vi "Read enemyGoalPosition.vi"(8 "error in (no error)":errorcluster, 11 "Field in":refnum<class "Field.lvclass">) -> (0 "error out":errorcluster, 2 "enemyGoalPosition":dbl[](array[numeric]), 3 "Field out":refnum<class "Field.lvclass">)   [LabVIEW 2020, in "Field.lvclass"]
uses:
  Field.lvclass
  Field.lvclass/Field.ctl
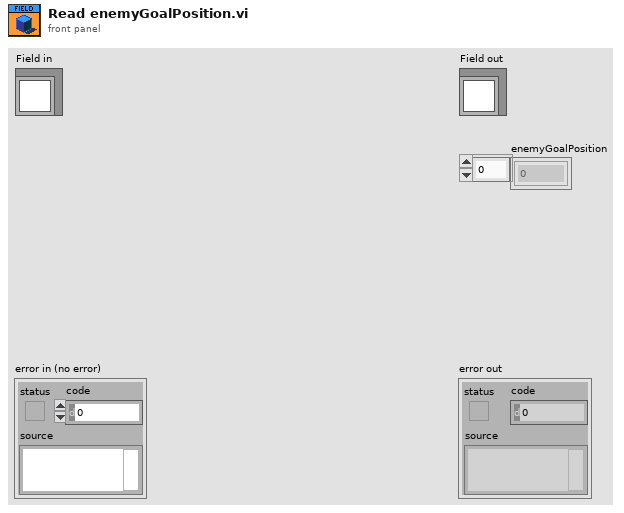
[diagram p1: front panel]
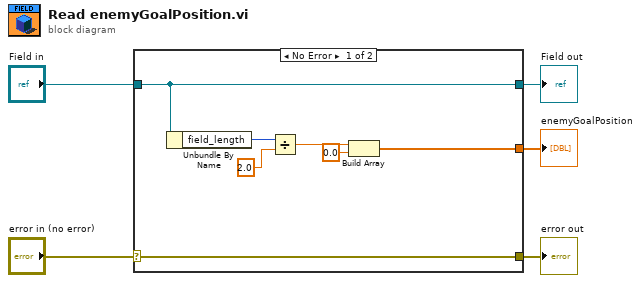
[diagram p0: block diagram]
diagram:
  n1 = case shown="No Error" "error in (no error)" {
    selector: "error in (no error)" -> [w12 w13]
    tunnel: [w12 w13] -> w4
    tunnel: [w11 w14] -> w2
    tunnel: "Field in" -> [w11 w14]
    tunnel: [w6 _] -> w1
    frame No Error {
      n2 = Unbundle By Name(w11) -> ("field_length"=w10:i32)
      n3 = Divide(x=w10, y=2.0) -> (x/y=w8:dbl)
      n4 = Build Array(w8, 0.0 ("element")) -> (w6:dbl[])
    }
    frame Error {
    }
  }
  "error out" <- w4
  "Field out" <- w2
  "enemyGoalPosition" <- w1
